vi "PADMINI_READ_ANALOG_DATA.vi"(11 "register values":u16[](array[numeric])) -> (3 "Array":i32[](array[numeric]))   [LabVIEW 2017]
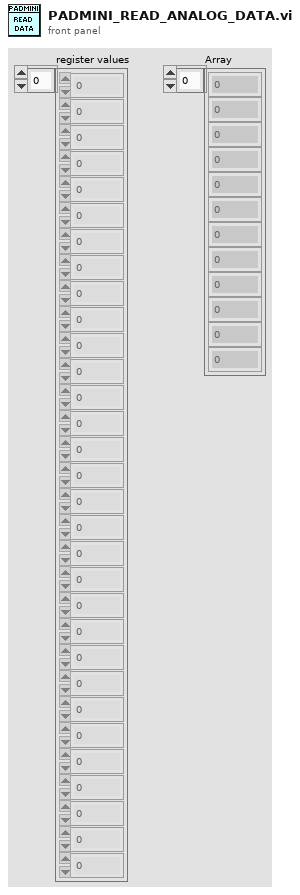
[diagram p1: front panel]
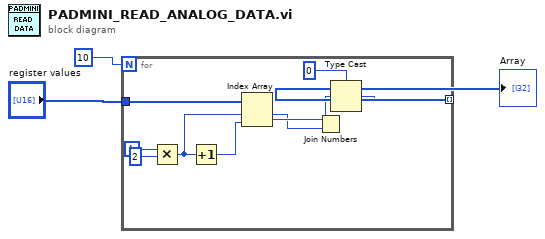
[diagram p0: block diagram]
diagram:
  n1 = for {
    N: 10 -> [_]
    tunnel: "register values" -> [w11]
    tunnel: [w12] -> w3 mode=indexing
    i -> [w10]
    n2 = Multiply(x=w10, y=2) -> (x*y=w8:i32)
    n3 = Increment(x=w8) -> (x+1=w7:i32)
    n4 = Index Array(array=w11, index #1=w8, index #2=w7) -> (element #1=w4:u16, element #2=w6:u16)
    n5 = Join Numbers(hi=w6, lo=w4) -> ((hi.lo)=w5:u32)
    n6 = Type Cast(type=0, x=w5) -> (*(type *) &x=w12:i32)
  }
  "Array" <- w3
